vi "Set Chopper Current.vi"(0 "Session Handle in":T1, 5 "RPM":u8, 11 "error in (no error)":errorcluster) -> (4 "Session Handle out":T1, 6 "Error Code":string, 15 "error out":errorcluster)   [LabVIEW 2015, in "PAS.lvclass"]
uses:
  PAS.lvclass
  Typedefs/Session Handle.ctl
panel:
  out "Success?":bool
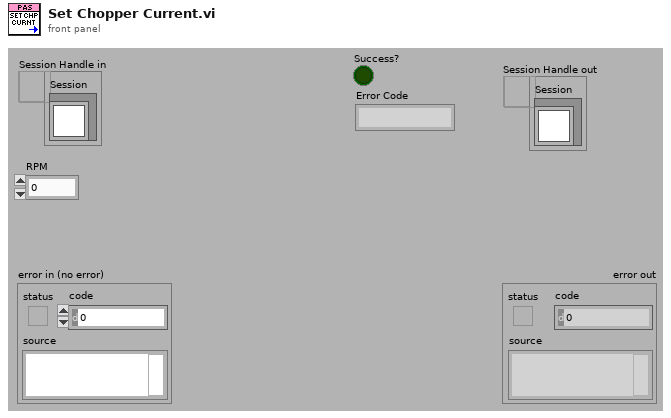
[diagram p1: front panel]
types:
  T1 = typedef "PAS.lvclass/Session Handle.ctl" = refnum<data-value>
  T2 = typedef "XNET Frame CAN.ctl" = cluster{"timestamp":timestamp, "payload":u8[], "identifier":u32, "type":T3, "extended?":bool, "echo?":bool}
  T3 = typedef "XNET Frame Type CAN.ctl" = u8
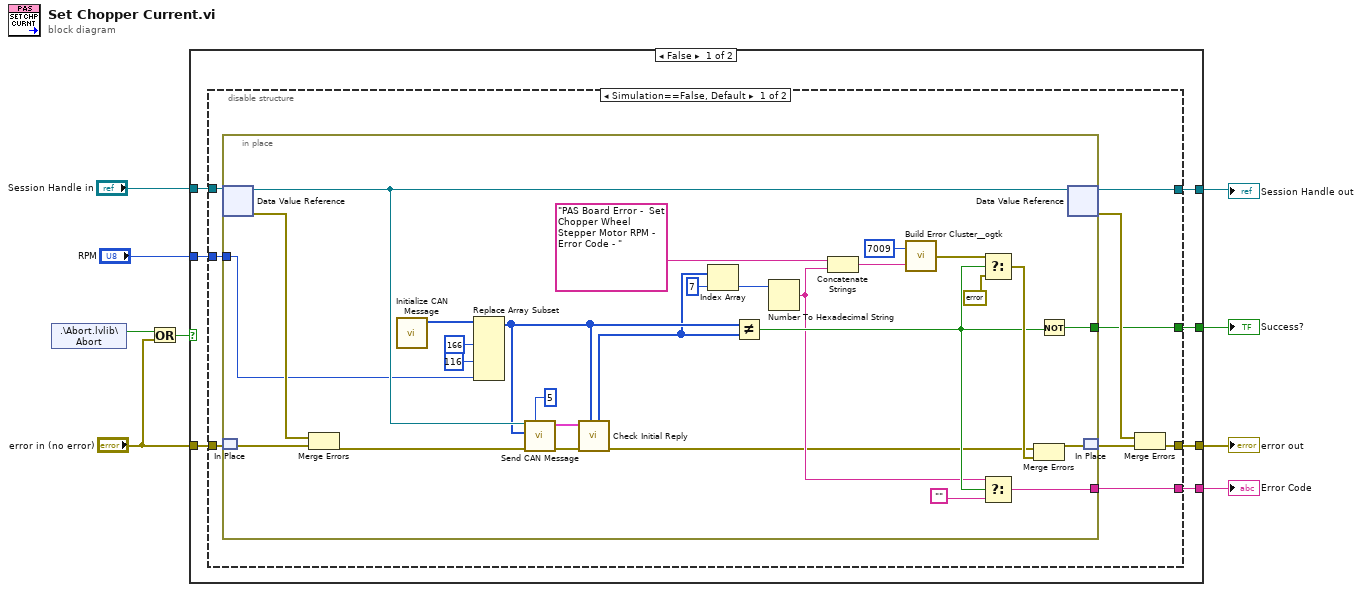
[diagram p0: block diagram]
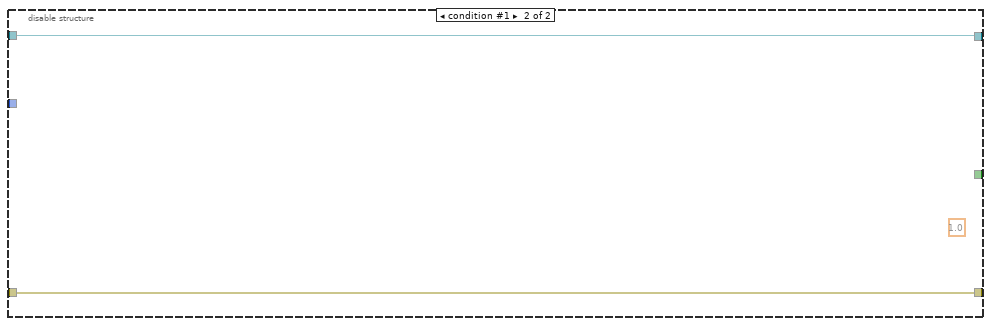
[diagram p2: hidden frame]
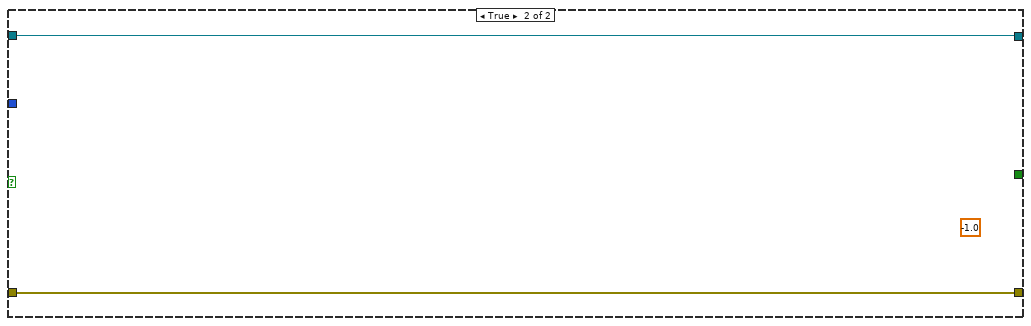
[diagram p3: hidden frame]
diagram:
  n1 = shared-variable ".\\Abort.lvlib\\Abort"() -> (w6:bool)  [unwired: 1 in, 1 out]
  n2 = Or(x=w6, y="error in (no error)") -> (x .or. y?=w4:bool)
  n3 = case shown="False" w4 {
    tunnel: [w16 w57] -> w8
    tunnel: [w15 w56] -> w7
    tunnel: "Session Handle in" -> [w14 w57]
    tunnel: "error in (no error)" -> [w13 w56]
    tunnel: [w12 _] -> w3
    tunnel: "RPM" -> [w11 _]
    tunnel: [w10 _] -> w1
    frame False {
      n4 = disable-structure shown="Simulation==False, Default" {
        disable-tunnel: [w25 w55] -> w16
        disable-tunnel: [w22 w54] -> w15
        disable-tunnel: w14 -> [w21 w55]
        disable-tunnel: w13 -> [w20 w54]
        disable-tunnel: [w19 _] -> w12
        disable-tunnel: w11 -> [w18 _]
        disable-tunnel: [w17 _] -> w10
        frame condition #0 (active) {
          n5 = in-place {
            in-place-border: [w43] -> w19
            in-place-border: w18 -> [w26]
            in-place-border: [w29] -> w17
            n6 = in-place-dvr #1(w21) -> (w46:refnum<class "PAS.lvclass">, w50:errorcluster)
            n7 = in-place-match #2(w20) -> (w49:errorcluster)
            n8 = Merge Errors(w50, w49) -> (w45:errorcluster)
            n9 = call "Initialize CAN Message.vi"() -> ("Initial Payload"=w51:u8[])  [unwired: 11 in]
            n10 = Replace Array Subset(array=w51, new element #1=u8 166 ("new element/subarray"), new element #2=u8 116 ("new element/subarray"), new element #3=w26) -> (w38:u8[])  [unwired: 3 in]
            n11 = call "Send CAN Message.vi"("Number of Retries"=5, "error in (no error)"=w45, "payload"=w38, "Gas In"=w46) -> ("error out"=w28:errorcluster, "Reply"=w47:T2[])  [unwired: 5 in, 1 out]
            n12 = call "Check Initial Reply.vi"("Write Message"=w38, "error in (no error)"=w28, "Reply"=w47) -> ("error out"=w27:errorcluster, "Whole Payload"=w37:u8[])  [unwired: 5 in, 2 out]
            n13 = Index Array(array=w37, index=7) -> (element=w35:u8)
            n14 = Not Equal?(x=w38, y=w37) -> (x != y?=w31:bool)
            n15 = Number To Hexadecimal String(2:w35) -> (0:w30:string)  [unwired: 1 in]
            n16 = Concatenate Strings("PAS Board Error -  Set Chopper Wheel Stepper Motor RPM - Error Code - " ("string"), w30) -> (w33:string)
            n17 = call <userlib>:"Build Error Cluster__ogtk.vi"("String to Prepend to source (\"\")"=w33, "code"=7009) -> ("error out"=w42:errorcluster)
            n18 = Select(t=w42, s=w31, f=errorcluster {"status"=FALSE, "code"=0, "source"=""}) -> (s? t:f=w39:errorcluster)
            n19 = Select(t=w30, s=w31, f="") -> (s? t:f=w29:string)
            n20 = Merge Errors(w27, w39) -> (w52:errorcluster)
            n21 = Not(x=w31) -> (.not. x?=w43:bool)
            n22 = in-place-dvr #1(w46) -> (w25:T1, w23:errorcluster)
            n23 = in-place-match #2(w52) -> (w24:errorcluster)
          }
          n24 = Merge Errors(w23, w24) -> (w22:errorcluster)
        }
        frame condition #1 {
          (unwired) 1.0
        }
      }
    }
    frame True {
      (unwired) -1.0
    }
  }
  "Session Handle out" <- w8
  "error out" <- w7
  "Success?" <- w3
  "Error Code" <- w1
